vi "Output.vi"(10 "Msg Output":refnum<class "Msg Output.lvclass">) -> ()   [LabVIEW 2025, in "_Template.lvlib" / "Templates.lvlib" / "TEMPLATE Msg.lvlib" / "TEMPLATE Msg Output.lvclass"]
uses:
  TEMPLATE Msg Output.lvclass
  jettl/jettl/Msg Output/Msg Output.lvclass
  TEMPLATE Msg Output.lvclass/TEMPLATE Msg Output.ctl
panel:
  # "This front panel should not be manipulated."
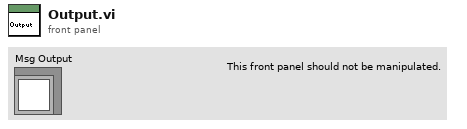
[diagram p1: front panel]
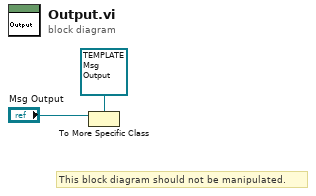
[diagram p0: block diagram]
diagram:
  # "This block diagram should not be manipulated."
  n1 = To More Specific Class(target class=refnum<class "TEMPLATE Msg Output.lvclass"> refnum ("_Template.lvlib:Templates.lvlib:TEMPLATE Msg.lvlib:TEMPLATE Msg Output.lvclass"), reference="Msg Output") -> ()  [unwired: 1 in, 2 out]
